vi "CAN Session.vi"(11 "interface":refnum<k21>) -> (1 "错误输出":errorcluster, 2 "read session":refnum<k21>, 3 "write session":refnum<k21>)   [LabVIEW 2018]
uses:
  <vilib>/xnet/xnet.llb/XNET Create Session (Frame Output Stream).vi
  <vilib>/xnet/xnet.llb/XNET Create Session (Frame Input Stream).vi
  <resource>/objmgr/xnet.rc
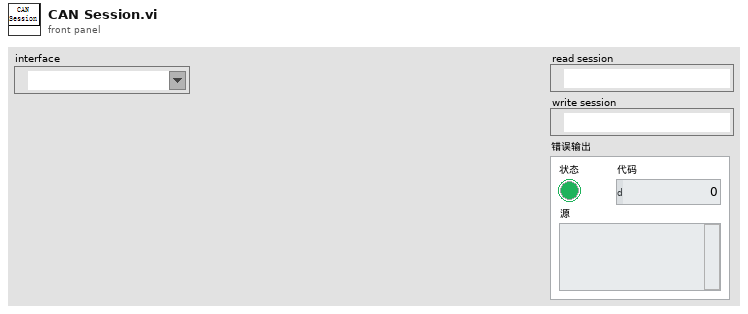
[diagram p1: front panel]
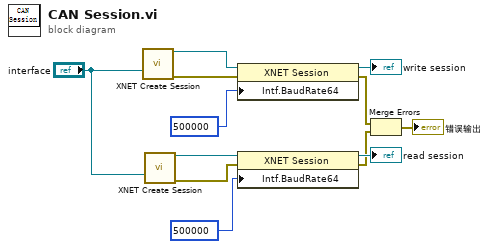
[diagram p0: block diagram]
diagram:
  n1 = call-poly <vilib>:"XNET Create Session.vi"("interface"="interface") -> ("session out"=w8:refnum<k21>, "error out"=w5:errorcluster)  [unwired: 13 in]
  n2 = call-poly <vilib>:"XNET Create Session.vi"("interface"="interface") -> ("session out"=w11:refnum<k21>, "error out"=w4:errorcluster)  [unwired: 13 in]
  n3 = property class="XNET Session"(reference=w8, error in=w5, "Intf.BaudRate64"=u64 500000 ("Interface:64bit Baud Rate")) -> (reference out=→"write session":refnum<k21>, error out=w3:errorcluster)
  n4 = property class="XNET Session"(reference=w11, error in=w4, "Intf.BaudRate64"=u64 500000 ("Interface:CAN:64bit FD Baud Rate")) -> (reference out=→"read session":refnum<k21>, error out=w2:errorcluster)
  n5 = Merge Errors(w3, w2) -> (→"错误输出":errorcluster)
